vi "merFISH_save_embryo_REF_position.vi"(4 "error in":errorcluster, 5 "queue ASI stage":refnum<queue>, 6 "ROI positions":dbl[][](array[numeric]), 7 "REF positions":dbl[][](array[numeric])) -> (0 "error out":errorcluster, 3 "REF positions OUT":dbl[][](array[numeric]))   [LabVIEW 2015]
uses:
  CONTROLS/Q_ASI_stage_element.ctl
  GLOBAL/Global_ASI_stage.vi
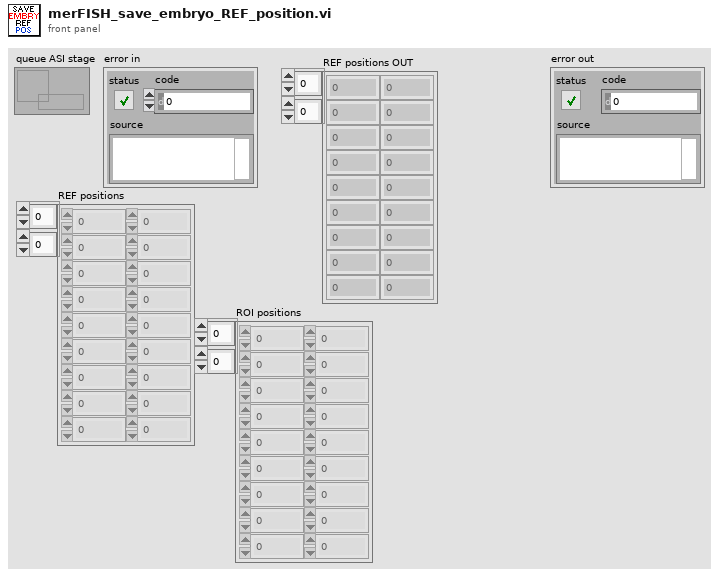
[diagram p1: front panel]
types:
  T1 = typedef "Q_ASI_stage_element.ctl" = cluster{"variant":variant, "Instruction":enum16{"ASI_idle", "ASI_initialize", "ASI_error", "ASI_security_stop", "ASI_read_XYZ", "ASI_up", "ASI_down", "ASI_left", "ASI_right", "ASI_save_XY", "ASI_move_to_XY", "ASI_brightfield", "ASI_init_scan", "ASI_init_merFISH", "ASI_move_to_XY_merFISH", "ASI_move_to_Z_merFISH", "ASI_init_autofocus_search_merFISH", "ASI_close_autofocus_search_merFISH", "ASI_adjust_piezo_autofocus_merFISH", "ASI_set_piezo_autofocus_to_reference_position_merFISH_TL", "ASI_close_merFISH", "ASI_stop"}}
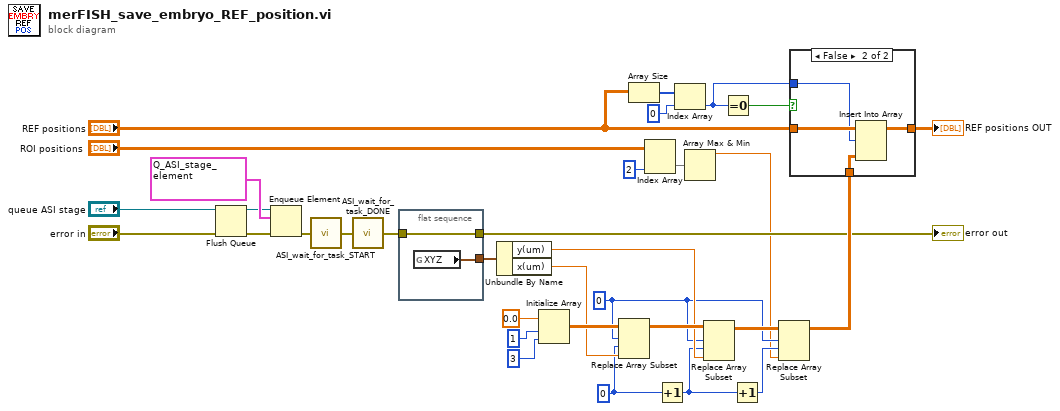
[diagram p0: block diagram]
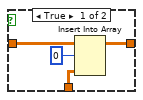
[diagram p2: hidden frame]
diagram:
  w13 = 0 ("index (row)")
  w14 = 0 ("index (row)")
  n1 = Flush Queue(queue="queue ASI stage", error in (no error)="error in") -> (queue out=w27:refnum<queue>, error out=w28:errorcluster)  [unwired: 1 out]
  n2 = Enqueue Element(queue=w27, element=T1 {"variant"=variant, "Instruction"=enum."ASI_save_XY"} ("Q_ASI_stage"), error in (no error)=w28) -> (error out=w30:errorcluster)  [unwired: 1 in, 2 out]
  n3 = call "ASI_wait_for_task_START.vi"("error in"=w30) -> ("error out"=w31:errorcluster)
  n4 = call "ASI_wait_for_task_DONE.vi"("error in"=w31) -> ("error out"=w32:errorcluster)
  n5 = flat-sequence {
    tunnel: w32 -> [w34]
    tunnel: [w35] -> w33
    tunnel: [w34] -> w3
    frame #0 {
      n6 = global read "Global_ASI_stage.vi" "XYZ"() -> (w35:cluster{"x(um)":dbl, "y(um)":dbl, "z(um)":dbl})
    }
  }
  n7 = Unbundle By Name(w33) -> ("y(um)"=w16:dbl, "x(um)"=w17:dbl)
  n8 = Initialize Array(0.0 ("element"), 1 ("dimension size"), 3 ("dimension size")) -> (w19:dbl[][])
  n9 = Replace Array Subset(array=w19, new element=w17, index (row)=w14, index (col)=w13) -> (w18:dbl[][])
  n10 = Array Size(array="REF positions") -> (size(s)=w8:i32[])
  n11 = Index Array(array="ROI positions", index (col)=2 ("disabled index (col)")) -> (element=w23:dbl[])  [unwired: 1 in]
  n12 = Increment(x=w13) -> (x+1=w12:i32)
  n13 = Index Array(array=w8, index=0) -> (element=w5:i32)
  n14 = Array Max & Min(array=w23) -> (max value=w2:dbl)  [unwired: 3 out]
  n15 = Replace Array Subset(array=w18, new element=w16, index (row)=w14, index (col)=w12) -> (w15:dbl[][])
  n16 = Equal To 0?(x=w5) -> (x = 0?=w4:bool)
  n17 = Increment(x=w12) -> (x+1=w11:i32)
  n18 = Replace Array Subset(array=w15, new element=w2, index (row)=w14, index (col)=w11) -> (w10:dbl[][])
  n19 = case shown="False" w4 {
    tunnel: w10 -> [w39 w43]
    tunnel: "REF positions" -> [w38 w42]
    tunnel: w5 -> [_ w40]
    tunnel: [w36 w41] -> w6
    frame True {
      n20 = Insert Into Array(array=w38, index (row)=0, new element=w39) -> (w36:dbl[][])  [unwired: 1 in]
    }
    frame False {
      n21 = Insert Into Array(array=w42, index (row)=w40, new element=w43) -> (w41:dbl[][])  [unwired: 1 in]
    }
  }
  "REF positions OUT" <- w6
  "error out" <- w3
